vi "AutoPlayParse.vi"(2 "Loaded Auto Play":string) -> (6 "Suggested Start Red":dbl[](array[numeric]), 7 "Full Auto Play Text":string, 8 "Suggested Start Blue":dbl[](array[numeric]), 9 "Documentation":string, 11 "Autonomous Path Suffix":string, 14 "Drive Command Strings":string[](array[string]), 15 "Drive Parameter Strings":string[](array[string]), 18 "Manipulator Command Strings":string[](array[string]), 19 "Manipulator Parameter Strings":string[](array[string]))   [LabVIEW 2023]
doc: "This VI parses a FRC 4265 standard autonomous play into two parallel sequences of steps and parameter strings. One sequence commands the robot's drive base while the other sequence commands the robot manipulator subsytems."
uses:
  GlobalDriverStationData.vi
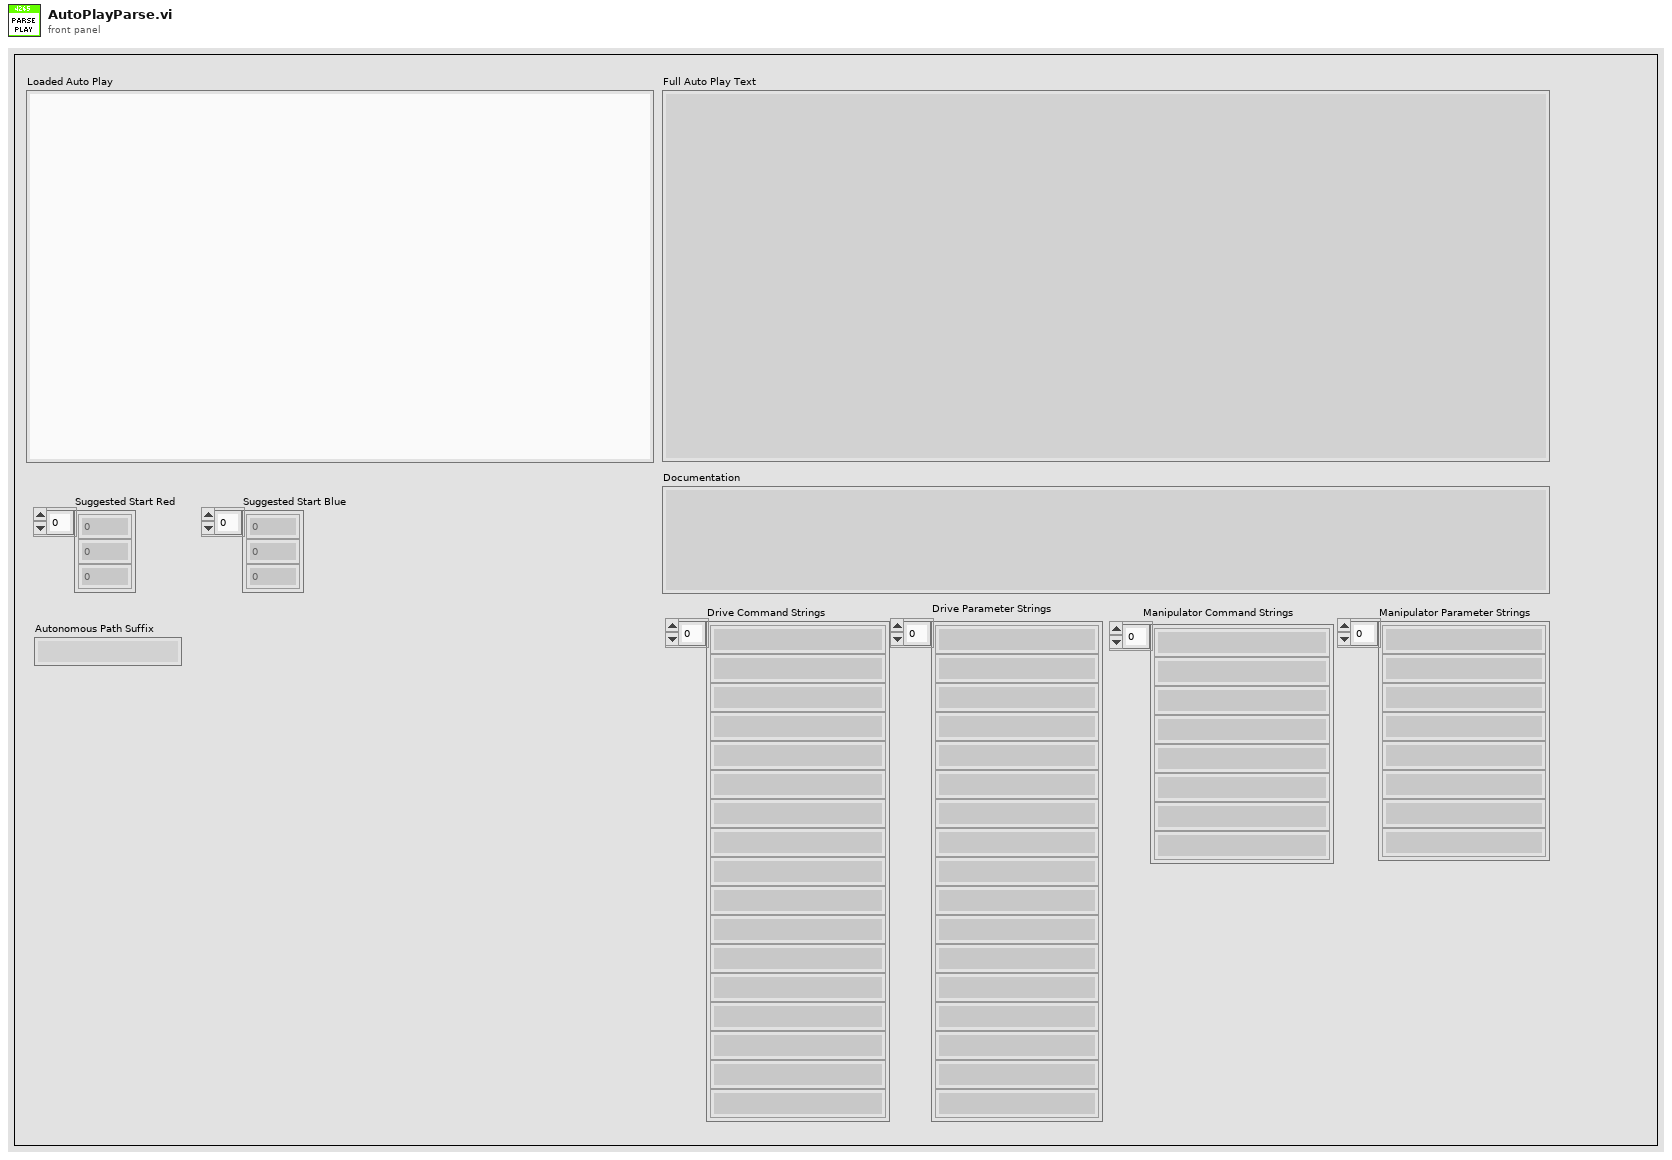
[diagram p1: front panel]
types:
  T1 = enum16{"Native", "Native Command Line", "UNIX", "Macintosh", "DOS"}
  T2 = typedef "WPI_DriverStationAllianceInfo.ctl" = enum16{"Red", "Blue", "Invalid"}
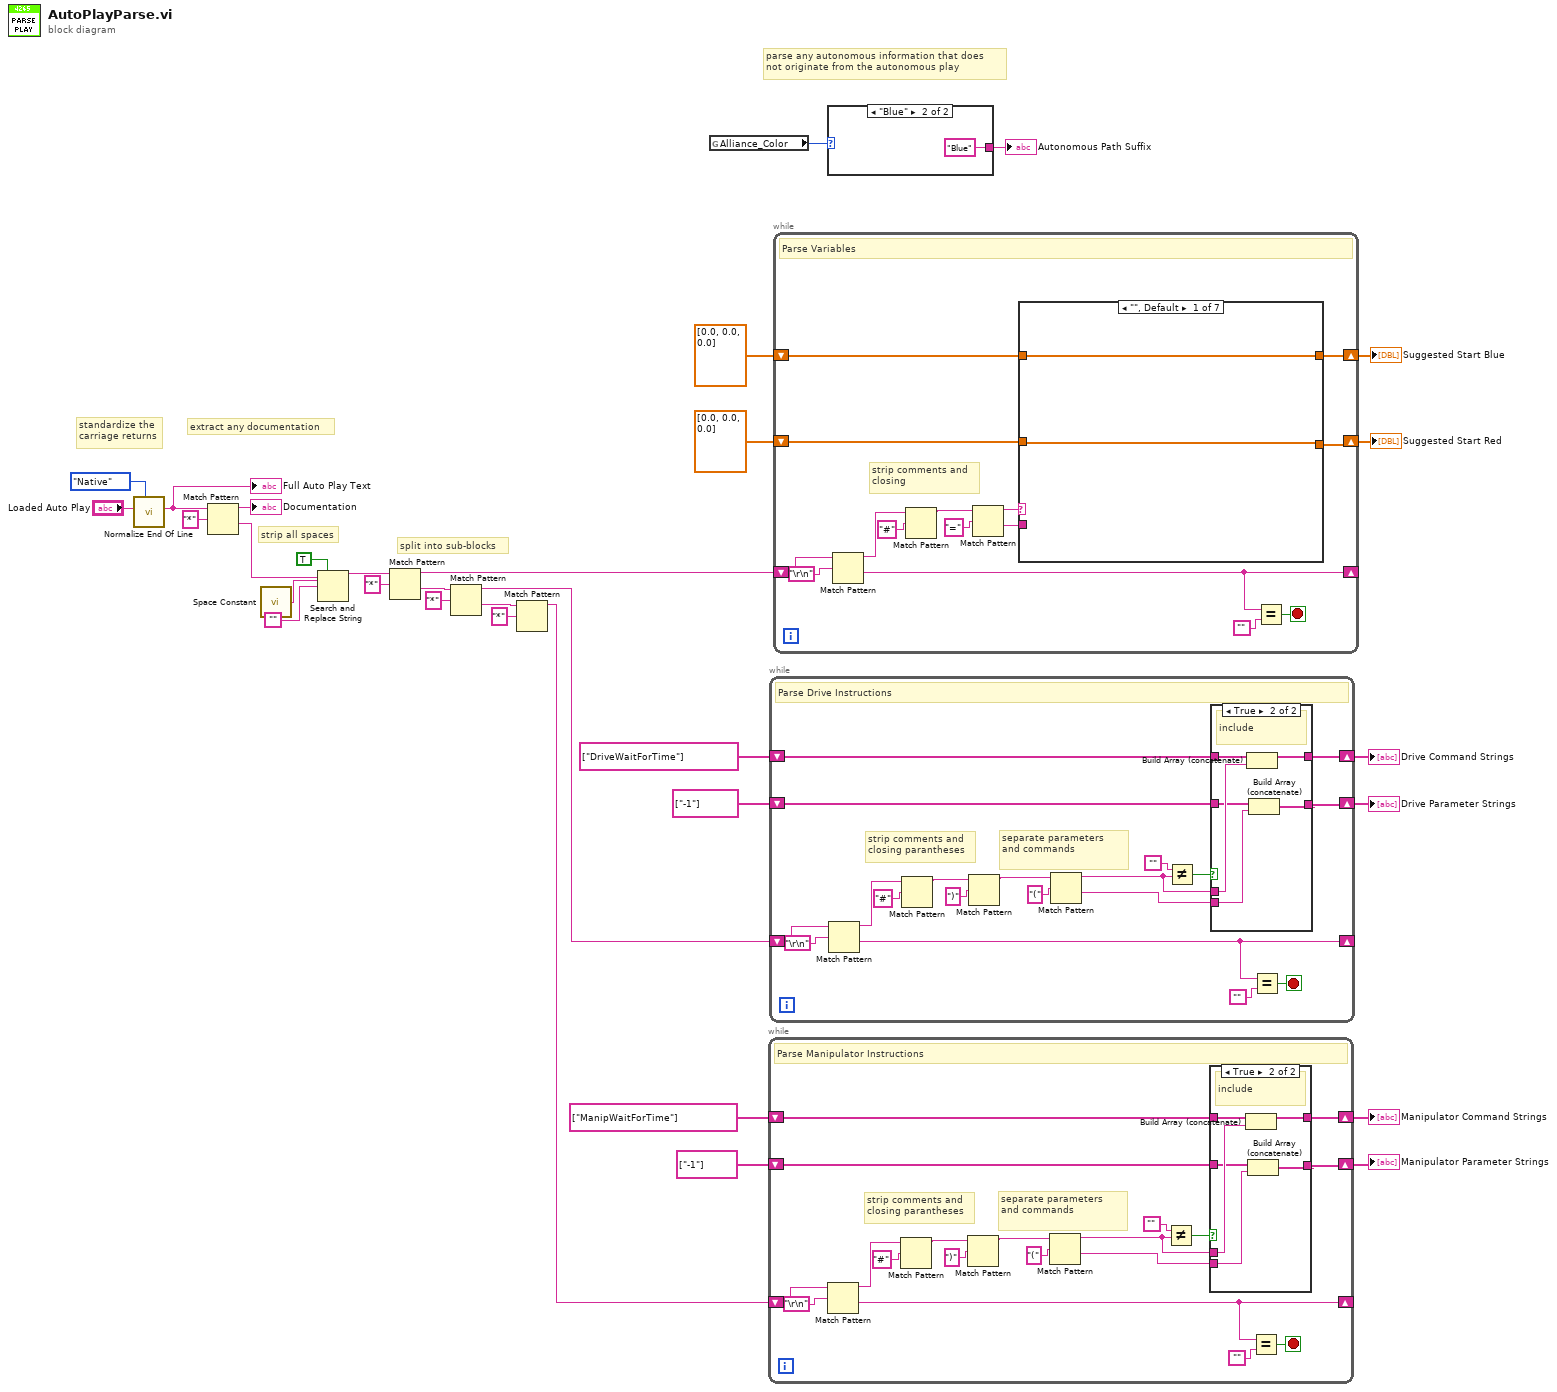
[diagram p0: block diagram]
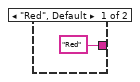
[diagram p2: hidden frame]
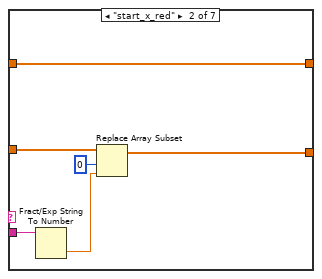
[diagram p3: hidden frame]
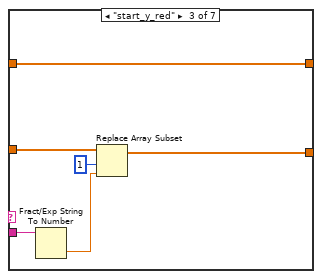
[diagram p4: hidden frame]
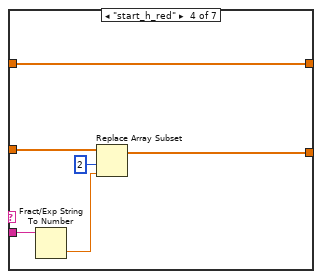
[diagram p5: hidden frame]
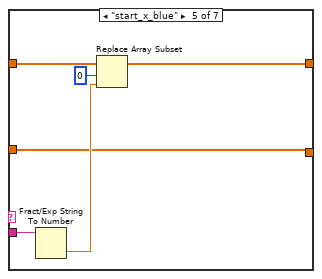
[diagram p6: hidden frame]
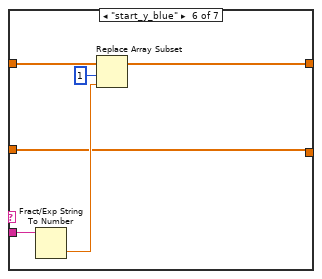
[diagram p7: hidden frame]
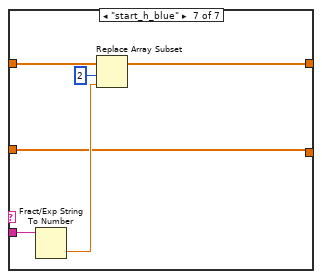
[diagram p8: hidden frame]
diagram:
  # "parse any autonomous information that does\nnot originate from the autonomous play"
  # "extract any documentation"
  # "split into sub-blocks"
  # "standardize the\ncarriage returns"
  # "strip all spaces"
  n1 = call <vilib>:"Normalize End Of Line.vi"("end of line (Native)"=T1."Native", "string in"="Loaded Auto Play") -> ("string out"=w16:string)  [unwired: 6 in]
  "Full Auto Play Text" <- w16
  n2 = Match Pattern(string=w16, regular expression="*") -> (before substring=→"Documentation":string, after substring=w19:string)  [unwired: 1 in, 2 out]
  n3 = call <vilib>:"Space Constant.vi"() -> ("String"=w28:string)
  n4 = Search and Replace String(replace all?=TRUE ("replace all? (F)"), input string=w19, search string=w28, replace string="") -> (result string=w8:string)  [unwired: 4 in, 3 out]
  n5 = Match Pattern(string=w8, regular expression="*") -> (before substring=w7:string, after substring=w9:string)  [unwired: 1 in, 2 out]
  n6 = Match Pattern(string=w9, regular expression="*") -> (before substring=w24:string, after substring=w25:string)  [unwired: 1 in, 2 out]
  n7 = Match Pattern(string=w25, regular expression="*") -> (before substring=w13:string)  [unwired: 1 in, 3 out]
  n8 = global read "GlobalDriverStationData.vi" "Alliance_Color"() -> (w2:T2)
  n9 = while {
    shift-right: [w35] -> _
    shift-left: w13 -> [w50]
    shift-right: [w36] -> w12
    shift-left: string[] ["ManipWaitForTime"] -> [w39]
    shift-right: [w37] -> w11
    shift-left: string[] ["-1"] -> [w38]
    stop <- w33 stop-if-true
    # "separate parameters\nand commands"
    # "strip comments and\nclosing parantheses"
    # "Parse Manipulator Instructions"
    n10 = Match Pattern(string=w50, regular expression="\r\n") -> (before substring=w46:string, after substring=w35:string)  [unwired: 1 in, 2 out]
    n11 = Match Pattern(string=w46, regular expression="#") -> (before substring=w47:string)  [unwired: 1 in, 3 out]
    n12 = Match Pattern(string=w47, regular expression=")") -> (before substring=w44:string)  [unwired: 1 in, 3 out]
    n13 = Match Pattern(string=w44, regular expression="(") -> (before substring=w41:string, after substring=w40:string)  [unwired: 1 in, 2 out]
    n14 = Not Equal?(x="", y=w41) -> (x != y?=w42:bool)
    n15 = case shown="True" w42 {
      tunnel: w41 -> [_ w58]
      tunnel: w40 -> [_ w56]
      tunnel: w39 -> [w53 w59]
      tunnel: w38 -> [w52 w57]
      tunnel: [w52 w55] -> w37
      tunnel: [w53 w54] -> w36
      frame False {
      }
      frame True {
        # "include"
        n16 = Build Array (concatenate)(w59, w58) -> (w54:string[])
        n17 = Build Array (concatenate)(w57, w56) -> (w55:string[])
      }
    }
    n18 = Equal?(x=w35, y="") -> (x = y?=w33:bool)
  }
  "Manipulator Parameter Strings" <- w11
  "Manipulator Command Strings" <- w12
  n19 = while {
    shift-right: [w62] -> _
    shift-left: w24 -> [w77]
    shift-right: [w63] -> w21
    shift-left: string[] ["DriveWaitForTime"] -> [w66]
    shift-right: [w64] -> w20
    shift-left: string[] ["-1"] -> [w65]
    stop <- w60 stop-if-true
    # "separate parameters\nand commands"
    # "strip comments and\nclosing parantheses"
    # "Parse Drive Instructions"
    n20 = Match Pattern(string=w77, regular expression="\r\n") -> (before substring=w73:string, after substring=w62:string)  [unwired: 1 in, 2 out]
    n21 = Match Pattern(string=w73, regular expression="#") -> (before substring=w74:string)  [unwired: 1 in, 3 out]
    n22 = Match Pattern(string=w74, regular expression=")") -> (before substring=w71:string)  [unwired: 1 in, 3 out]
    n23 = Match Pattern(string=w71, regular expression="(") -> (before substring=w68:string, after substring=w67:string)  [unwired: 1 in, 2 out]
    n24 = Not Equal?(x="", y=w68) -> (x != y?=w69:bool)
    n25 = case shown="True" w69 {
      tunnel: w68 -> [_ w85]
      tunnel: w67 -> [_ w83]
      tunnel: w66 -> [w80 w86]
      tunnel: w65 -> [w79 w84]
      tunnel: [w79 w82] -> w64
      tunnel: [w80 w81] -> w63
      frame False {
      }
      frame True {
        # "include"
        n26 = Build Array (concatenate)(w86, w85) -> (w81:string[])
        n27 = Build Array (concatenate)(w84, w83) -> (w82:string[])
      }
    }
    n28 = Equal?(x=w62, y="") -> (x = y?=w60:bool)
  }
  "Drive Parameter Strings" <- w20
  "Drive Command Strings" <- w21
  n29 = while {
    shift-right: [w95] -> _
    shift-left: w7 -> [w100]
    shift-right: [w89] -> w3
    shift-left: dbl[] [0.0, 0.0, 0.0] -> [w90]
    shift-right: [w87] -> w4
    shift-left: dbl[] [0.0, 0.0, 0.0] -> [w88]
    stop <- w93 stop-if-true
    # "strip comments and\nclosing"
    # "Parse Variables"
    n30 = Match Pattern(string=w100, regular expression="\r\n") -> (before substring=w96:string, after substring=w95:string)  [unwired: 1 in, 2 out]
    n31 = Match Pattern(string=w96, regular expression="#") -> (before substring=w97:string)  [unwired: 1 in, 3 out]
    n32 = Match Pattern(string=w97, regular expression="=") -> (before substring=w91:string, after substring=w92:string)  [unwired: 1 in, 2 out]
    n33 = case shown="\"\", Default" w91 {
      tunnel: w92 -> [_ w109 w115 w121 w127 w133 w139]
      tunnel: w90 -> [w102 w108 w114 w120 w122 w128 w134]
      tunnel: [w102 w105 w111 w117 w122 w128 w134] -> w89
      tunnel: w88 -> [w103 w104 w110 w116 w124 w130 w136]
      tunnel: [w103 w104 w110 w116 w123 w129 w135] -> w87
      frame "", Default {
      }
      frame "start_x_red" {
        # "include"
        n34 = Fract/Exp String To Number(string=w109) -> (number=w106:dbl)  [unwired: 3 in, 1 out]
        n35 = Replace Array Subset(array=w108, new element=w106, index=0) -> (w105:dbl[])
      }
      frame "start_y_red" {
        # "include"
        n36 = Fract/Exp String To Number(string=w115) -> (number=w112:dbl)  [unwired: 3 in, 1 out]
        n37 = Replace Array Subset(array=w114, new element=w112, index=1) -> (w111:dbl[])
      }
      frame "start_h_red" {
        # "include"
        n38 = Fract/Exp String To Number(string=w121) -> (number=w118:dbl)  [unwired: 3 in, 1 out]
        n39 = Replace Array Subset(array=w120, new element=w118, index=2) -> (w117:dbl[])
      }
      frame "start_x_blue" {
        # "include"
        n40 = Fract/Exp String To Number(string=w127) -> (number=w125:dbl)  [unwired: 3 in, 1 out]
        n41 = Replace Array Subset(array=w124, new element=w125, index=0) -> (w123:dbl[])
      }
      frame "start_y_blue" {
        # "include"
        n42 = Fract/Exp String To Number(string=w133) -> (number=w131:dbl)  [unwired: 3 in, 1 out]
        n43 = Replace Array Subset(array=w130, new element=w131, index=1) -> (w129:dbl[])
      }
      frame "start_h_blue" {
        # "include"
        n44 = Fract/Exp String To Number(string=w139) -> (number=w137:dbl)  [unwired: 3 in, 1 out]
        n45 = Replace Array Subset(array=w136, new element=w137, index=2) -> (w135:dbl[])
      }
    }
    n46 = Equal?(x=w95, y="") -> (x = y?=w93:bool)
  }
  "Suggested Start Blue" <- w4
  "Suggested Start Red" <- w3
  n47 = case shown="\"Blue\"" w2 {
    tunnel: ["Red" ("refnum name") "Blue" ("refnum name")] -> w1
    frame "Red", Default {
    }
    frame "Blue" {
    }
  }
  "Autonomous Path Suffix" <- w1
